vi "DemandedPositionAdjustment.vi"(7 "Extra Command String":string, 9 "Simulate/Run":T1, 11 "Demanded Position":sgl[](array[numeric])) -> (3 "Adjusted Position":sgl[](array[numeric]))   [LabVIEW 2015]
uses:
  Controls/User_Specific_mode.ctl
  Globals/Extra_Commands_Global.vi
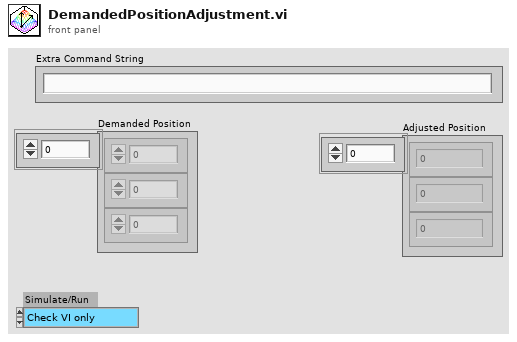
[diagram p1: front panel]
types:
  T1 = typedef "User_Specific_mode.ctl" = enum16{"Check VI only", "Run VI"}
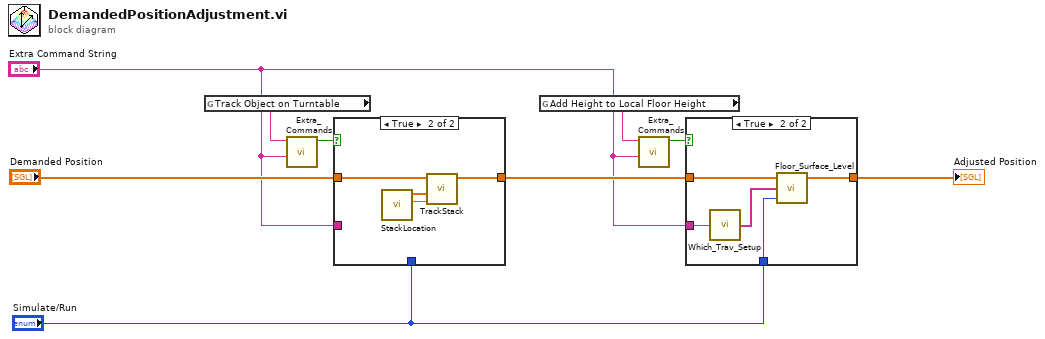
[diagram p0: block diagram]
diagram:
  n1 = global read "Extra_Commands_Global.vi" "Track Object on Turntable"() -> (w6:string)
  n2 = call "Extra_Commands.vi"("String to Search"="Extra Command String", "Command"=w6) -> ("Command Found"=w5:bool)  [unwired: 1 in, 4 out]
  n3 = case shown="True" w5 {
    tunnel: "Demanded Position" -> [w10 w14]
    tunnel: [w10 w13] -> w3
    tunnel: "Simulate/Run" -> [_ _]
    tunnel: "Extra Command String" -> [_ _]
    frame False {
    }
    frame True {
      n4 = call "StackLocation.vi"() -> ("Current\nWindDirection"=w11:dbl, "StackPosition (at 0deg)"=w12:sgl[])  [unwired: 10 in]
      n5 = call "TrackStack.vi"("WindDirection"=w11, "StackPosition (at 0deg)"=w12, "Demanded Position"=w14) -> ("Adjusted Position"=w13:sgl[])  [unwired: 7 in, 1 out]
    }
  }
  n6 = global read "Extra_Commands_Global.vi" "Add Height to Local Floor Height"() -> (w7:string)
  n7 = call "Extra_Commands.vi"("String to Search"="Extra Command String", "Command"=w7) -> ("Command Found"=w8:bool)  [unwired: 1 in, 4 out]
  n8 = case shown="True" w8 {
    tunnel: w3 -> [w15 w20]
    tunnel: [w15 w19] -> w9
    tunnel: "Simulate/Run" -> [_ w18]
    tunnel: "Extra Command String" -> [_ w17]
    frame False {
    }
    frame True {
      n9 = call "Which_Trav_Setup.vi"("Extra Command String"=w17) -> ("Traverse Setups"=w16:string[])
      n10 = call "Floor_Surface_Level.vi"("Simulate/Run"=w18, "Traverse Setups"=w16, "Position In"=w20) -> ("Position Out"=w19:sgl[])  [unwired: 2 out]
    }
  }
  "Adjusted Position" <- w9
